vi "Project-Milestone-3.vi"() -> ()   [LabVIEW 2010]
uses:
  <vilib>/ptbypt/NI_PtbyPt.lvlib
panel:
  out "Distance":dbl(graph)
  out "Duty Cycle":dbl(graph)
  out "Distance \n 2":dbl format="%#_3g"
  out "Distance":dbl(knob) scale=5.0..11.0 scale format="%#_2g"
  out "Voltage":dbl format="%#_4g"
  out "Mean":dbl(graph)
  out "Filter":dynamicdata(graph)
  in  "Sample Rate":dbl=1000.0
  in  "Number of Samples to Read":i32=100
  out "Signal":dynamicdata(graph)
  in  "stop 2":bool
  in  "stop":bool
  out "Position Error":dbl format="%#_4g"
  out "Direction":bool
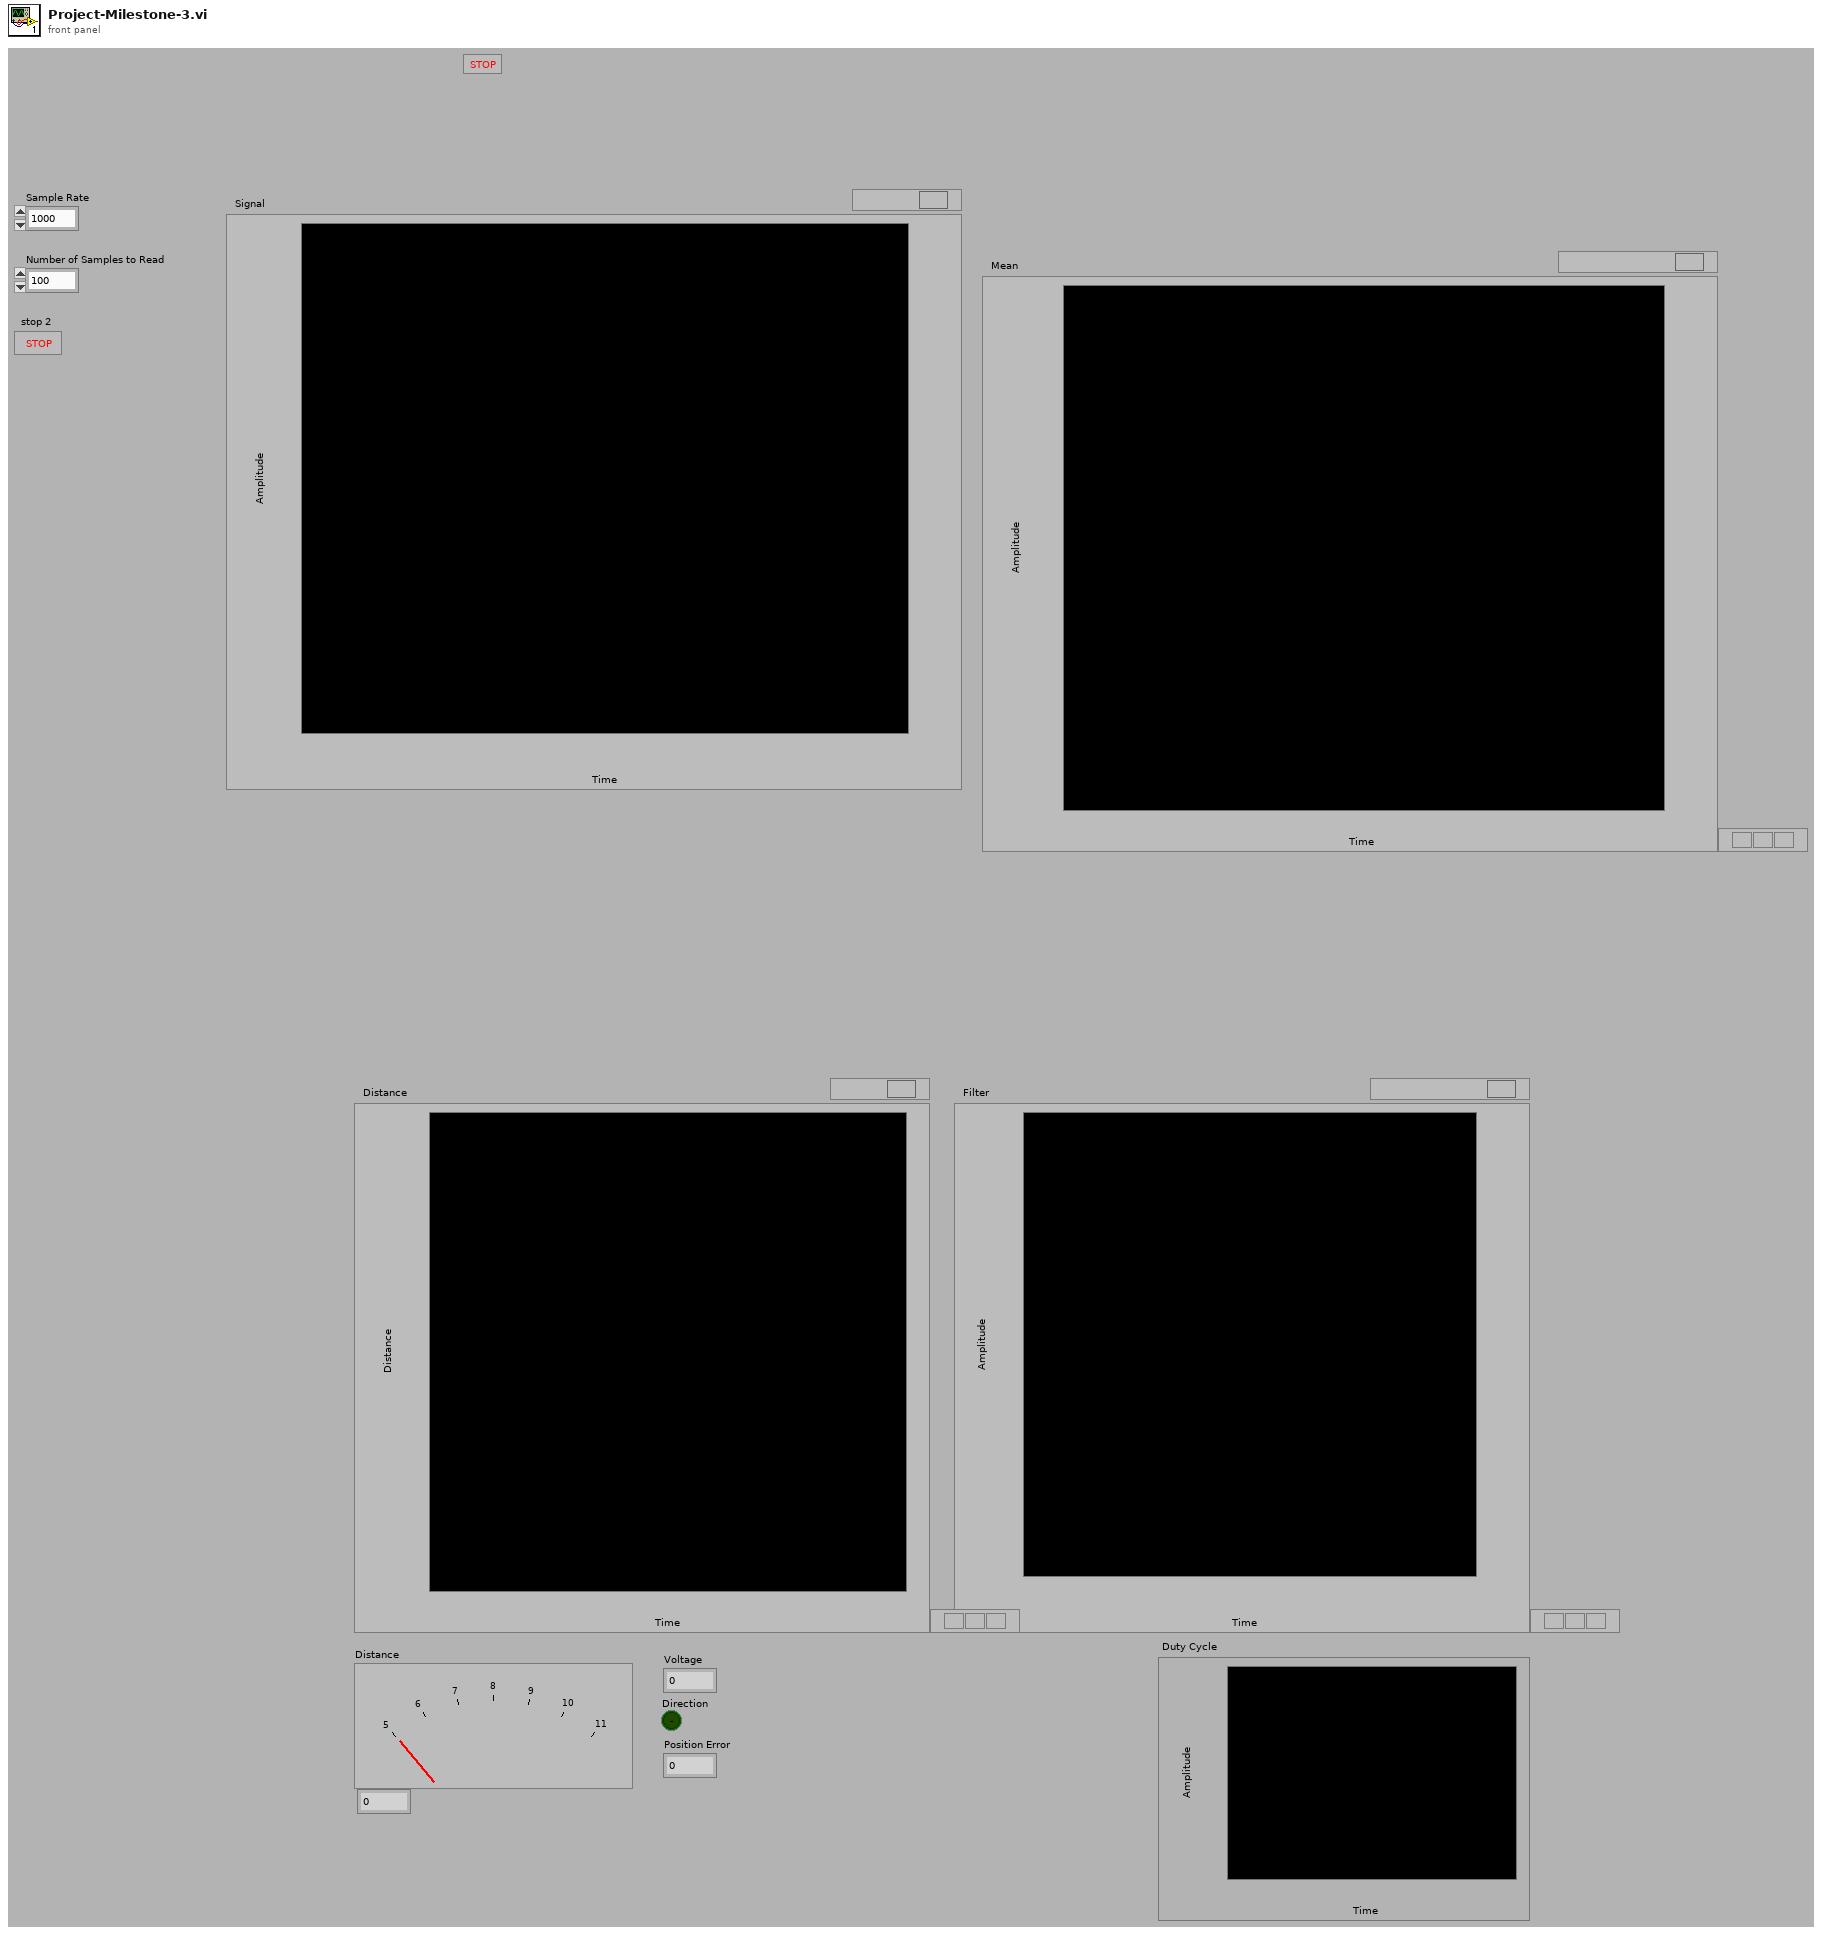
[diagram p1: front panel]
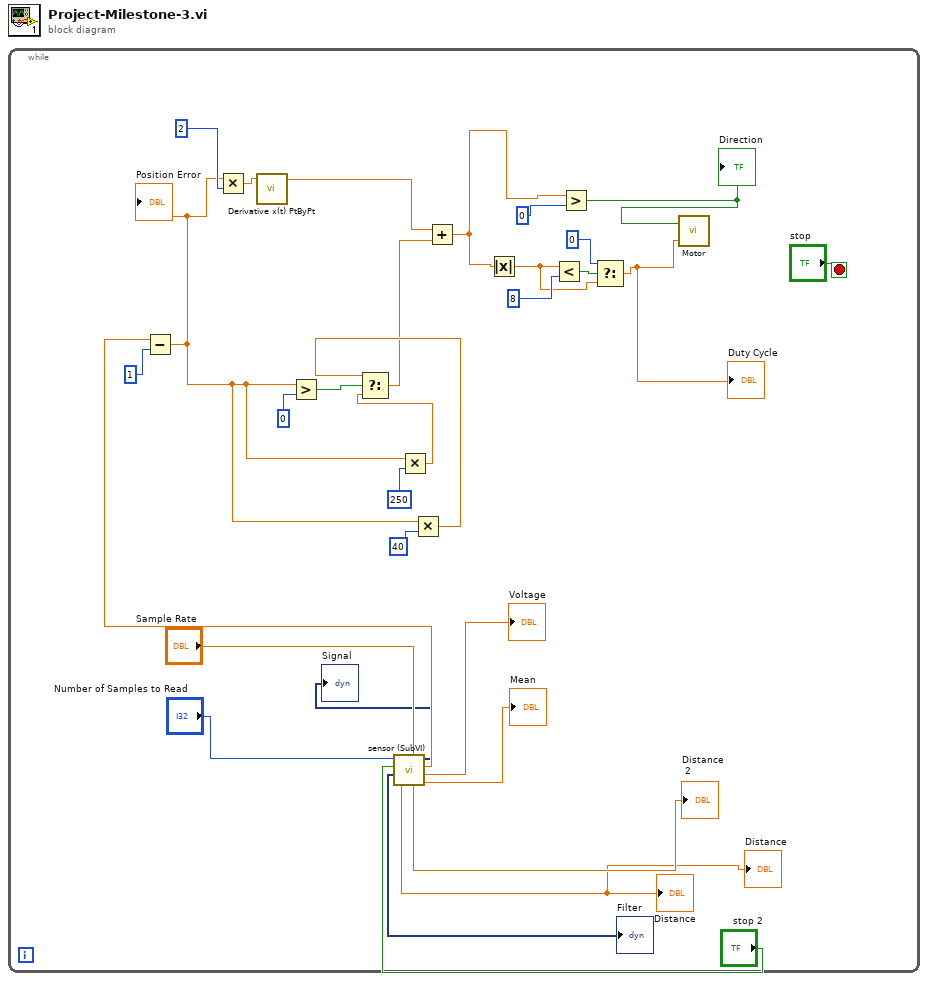
[diagram p0: block diagram]
diagram:
  n1 = while {
    stop <- "stop" stop-if-true
    n2 = call "sensor (SubVI).vi"("stop 2"="stop 2", "Number of Samples to Read"="Number of Samples to Read", "Sample Rate"="Sample Rate") -> ("Distance"=→"Distance" →"Distance":dbl, "Filter"=→"Filter":dynamicdata, "Distance \n 2"=→"Distance \n 2":dbl, "Mean"=→"Mean":dbl, "Voltage"=→"Voltage":dbl, "Result"=w25:dbl, "Signal"=→"Signal":dynamicdata)
    n3 = Subtract(x=w25, y=1) -> (x-y=w11:dbl)
    "Position Error" <- w11
    n4 = Multiply(x=w11, y=2) -> (x*y=w20:dbl)
    n5 = call <vilib>:"Derivative x(t) PtByPt.vi"("x"=w20) -> ("dx/dt"=w24:dbl)  [unwired: 3 in, 1 out]
    n6 = Greater?(x=w11, y=0) -> (0:w14:bool)
    n7 = Multiply(x=w11, y=250) -> (x*y=w10:dbl)
    n8 = Multiply(x=w11, y=40) -> (x*y=w13:dbl)
    n9 = Select(t=w13, s=w14, f=w10) -> (s? t:f=w9:dbl)
    n10 = Add(x=w24, y=w9) -> (x+y=w22:dbl)
    n11 = Absolute Value(x=w22) -> (abs(x)=w2:dbl)
    n12 = Less?(x=w2, y=8) -> (x < y?=w5:bool)
    n13 = Greater?(x=w22, y=0) -> (0:w31:bool)
    "Direction" <- w31
    n14 = Select(t=0, s=w5, f=w2) -> (s? t:f=w3:dbl)
    "Duty Cycle" <- w3
    n15 = call "Motor.vi"("Duty Cycle (%) 2"=w3, "Motor Dir 2"=w31) -> ()  [unwired: 1 out]
  }
